vi "[Template]_Read.vi"(8 "error in (no error)":errorcluster, 9 "Default":T1, 11 "Tag Name":string) -> (0 "error out":errorcluster, 1 "Data":T1)   [LabVIEW 2016]
doc: "This VI will read the data associated with a single tag. This VI will always look up the tag index if the name changes, or if index lookup failed previously (resulting in an error). This combines the functionality of the CVT2 VIs for reads and static reads."
uses:
  <vilib>/NI/Current Value Table/DataTypes/[Template]_Datatype.ctl
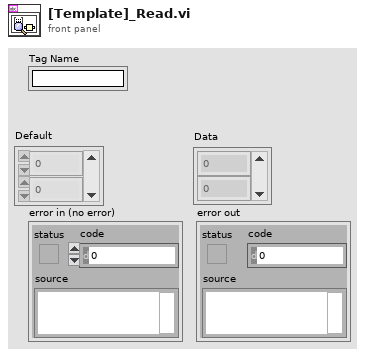
[diagram p1: front panel]
types:
  T1 = typedef "[Template]_Datatype.ctl" = i32[]
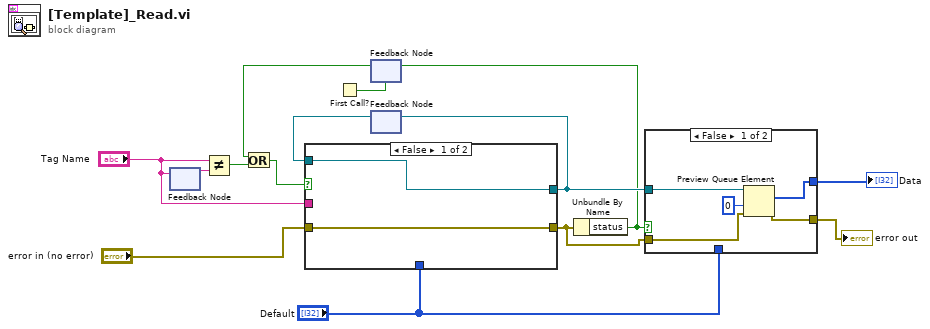
[diagram p0: block diagram]
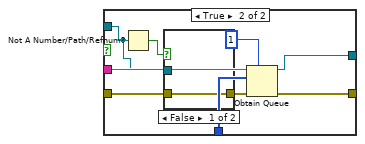
[diagram p3: hidden frame]
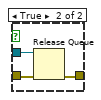
[diagram p4: hidden frame]
diagram:
  n1 = feedback #1() -> (w13:string)  [unwired: 1 in]
  n2 = feedback-in #1("Tag Name") -> ()
  n3 = Not Equal?(x="Tag Name", y=w13) -> (x != y?=w9:bool)
  n4 = First Call?() -> (First Call?: T/F=w5:bool)
  n5 = feedback #2(w5) -> (w7:bool)
  n6 = Or(x=w7, y=w9) -> (x .or. y?=w6:bool)
  n7 = feedback #3() -> (w12:refnum<queue>)  [unwired: 1 in]
  n8 = case shown="False" w6 {
    tunnel: [w16 w25] -> w2
    tunnel: "error in (no error)" -> [w16 w18]
    tunnel: [w15 w24] -> w11
    tunnel: w12 -> [w15 w19]
    tunnel: "Default" -> [_ w21]
    tunnel: "Tag Name" -> [_ w23]
    frame False {
    }
    frame True {
      n9 = Not A Number/Path/Refnum?(number/path/refnum=w19) -> (NaN/Path/Refnum?=w20:bool)
      n10 = case shown="False" w20 {
        tunnel: w18 -> [w26 w28]
        tunnel: [w26 w29] -> w17
        tunnel: w19 -> [_ w27]
        frame False {
        }
        frame True {
          n11 = Release Queue(queue=w27, error in (no error)=w28) -> (error out=w29:errorcluster)  [unwired: 1 in, 2 out]
        }
      }
      n12 = Obtain Queue(max queue size (-1, unlimited)=1, name (unnamed)=w23, element data type=w21, error in (no error)=w17) -> (queue out=w24:refnum<queue>, error out=w25:errorcluster)  [unwired: 1 in, 1 out]
    }
  }
  n13 = feedback-in #3(w11) -> ()
  n14 = Unbundle By Name(w2) -> ("status"=w8:bool)
  n15 = feedback-in #2(w8) -> ()
  n16 = case shown="False" w8 {
    tunnel: w11 -> [w34 _]
    tunnel: "Default" -> [_ w36]
    tunnel: [w30 w36] -> w3
    tunnel: w2 -> [w32 w35]
    tunnel: [w31 w35] -> w1
    frame False {
      n17 = Preview Queue Element(queue=w34, timeout in ms (-1)=0, error in (no error)=w32) -> (element=w30:T1, error out=w31:errorcluster)  [unwired: 2 out]
    }
    frame True {
    }
  }
  "error out" <- w1
  "Data" <- w3
